vi "DSF.Engine.Pool.Get Debug Flags.vi"(11 "Pool in":refnum<class "DSF.Engine.Pool.lvclass">) -> (2 "FIFO Debug Flags":refnum<class "Debug Flags FIFO.lvclass">, 3 "Pool out":refnum<class "DSF.Engine.Pool.lvclass">)   [LabVIEW 2017, in "Data Sharing Framework Engine.lvlib" / "DSF.Engine.Pool.lvclass"]
uses:
  DSF.Engine.Pool.lvclass
  Source/Data Sharing Framework Core/Engine/Debug/Debug Flags FIFO/Debug Flags FIFO.lvclass
  DSF.Engine.Pool.lvclass/DSF.Engine.Pool.ctl
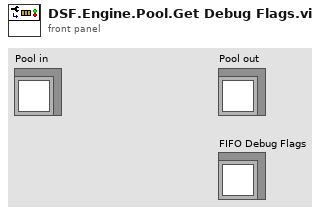
[diagram p1: front panel]
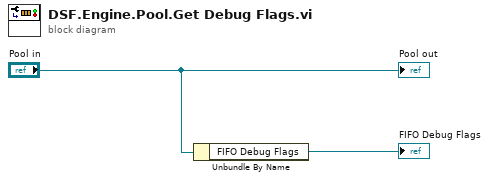
[diagram p0: block diagram]
diagram:
  n1 = Unbundle By Name("Pool in") -> ("FIFO Debug Flags"=→"FIFO Debug Flags":refnum<class "Debug Flags FIFO.lvclass">)
  "Pool out" <- "Pool in"
